vi "Test Warning Dialog.vi"(4 "error in (no error)":errorcluster, 7 "Warning Message":string) -> (0 "error out":errorcluster)   [LabVIEW 2011]
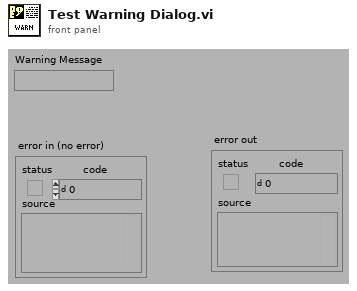
[diagram p1: front panel]
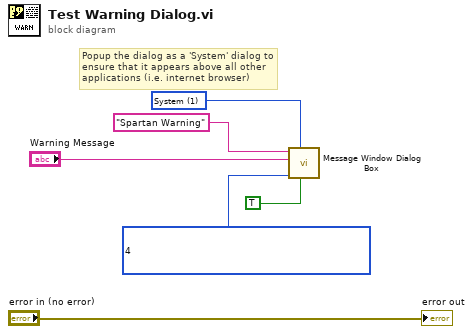
[diagram p0: block diagram]
diagram:
  w5 = 1 items=["Application", "System", "Task"] ("modality (0)")
  # "Popup the dialog as a 'System' dialog to ensure that it appears above all other applications (i.e. internet browser)"
  n1 = call "Message Window Dialog Box.vi"("sound? (F)"=TRUE, "modality (0)"=w5, "icon (0:None)"=4, "message (\"\")"="Warning Message", "window title (\"\")"="Spartan Warning" ("window title (\"\")")) -> ()  [unwired: 2 in, 4 out]
  "error out" <- "error in (no error)"
